vi "Get Camera FOV.vi"() -> ()   [LabVIEW 2015]
uses:
  Camera Types2.ctl
panel:
  in  "Camera Type2":T1
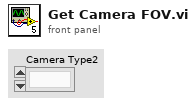
[diagram p1: front panel]
types:
  T1 = typedef "Camera Types2.ctl" = enum16{""}
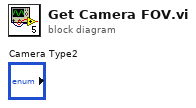
[diagram p0: block diagram]
diagram:
